vi "MtAtElectrometer_acceptCommand_performZeroCalib.vi"(8 "error in (no error)":errorcluster, 11 "command_performZeroCalib_Ctl":T1) -> (0 "error out":errorcluster, 2 "function return":i32, 3 "command_performZeroCalib_Ctl out":T1)   [LabVIEW 2016, in "SALLV_MtAtElectrometer.lvlib"]
doc: "int MtAtElectrometer_shm_acceptCommand_performZeroCalibLV(MtAtElectrometer_command_performZeroCalibLV *command_performZeroCalib_Ctl );"
uses:
  SALLV_MtAtElectrometer.lvlib
  DataTypes/command_performZeroCalib.ctl
  ts_sal/test/MtAtElectrometer/labview/SALLV_MtAtElectrometer.so
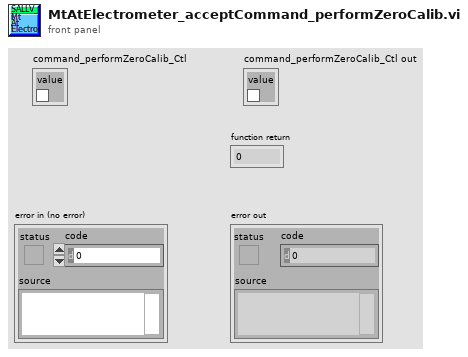
[diagram p1: front panel]
types:
  T1 = typedef "SALLV_MtAtElectrometer.lvlib/command_performZeroCalib.ctl" = cluster{"value":bool}
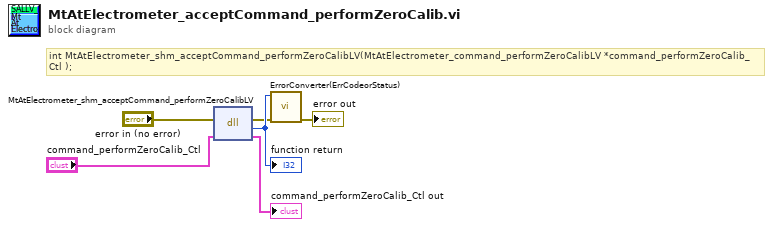
[diagram p0: block diagram]
diagram:
  # "int MtAtElectrometer_shm_acceptCommand_performZeroCalibLV(MtAtElectrometer_command_performZeroCalibLV *command_performZeroCalib_Ctl );"
  n1 = dll-call lib="home/andres/ts_sal/test/MtAtElectrometer/labview/SALLV_MtAtElectrometer.*" fn="MtAtElectrometer_shm_acceptCommand_performZeroCalibLV"(error in="error in (no error)", "command_performZeroCalib_Ctl"="command_performZeroCalib_Ctl") -> (error out=w2:errorcluster, w6:i32, "command_performZeroCalib_Ctl"=→"command_performZeroCalib_Ctl out":T1)  [unwired: 2 in, 1 out]
  "function return" <- w6
  n2 = call "ErrorConverter(ErrCodeorStatus).vi"("error in (no error)"=w2, "error code"=w6) -> ("error out"=→"error out":errorcluster)  [unwired: 9 in]
